vi "CRYAcq Get Channel Name.vi"(0 "I_channel Info Out":T2[](array[typedef]) {"Coupling" items=["Default"=-1, "RSE"=10083, "NRSE"=10078, "Differential"=10106, "Pseudodifferential"=12529]; "term config" items=["Default"=-1, "RSE"=10083, "NRSE"=10078, "Differential"=10106, "Pseudodifferential"=12529]; "Anti-aliasing Factor (%fs)" format="%.2f"}, 1 "O_channel Info Out":T2[](array[typedef]) {"Coupling" items=["Default"=-1, "RSE"=10083, "NRSE"=10078, "Differential"=10106, "Pseudodifferential"=12529]; "term config" items=["Default"=-1, "RSE"=10083, "NRSE"=10078, "Differential"=10106, "Pseudodifferential"=12529]; "Anti-aliasing Factor (%fs)" format="%.2f"}, 5 "Cluster":cluster{"RecDeviceID":u32, "Audio Driver":u32}, 9 "RecChannel":u16, 11 "Selected Play In":string[][](array[string]), 12 "Index for testinfor":i32, 13 "Acquisition Type":T1(ring)) -> (3 "Vmax In":dbl, 4 "ChannelName In":string caption="ChannelName", 6 "Test Info":string, 10 "Play Channel Name":string, 14 "In data Len":i32, 15 "Latency (samples) In":dbl)   [LabVIEW 2013]
uses:
  Typedef Control/CRYHardware Channel Info.ctl
panel:
  out "subarray":string[](array[string])
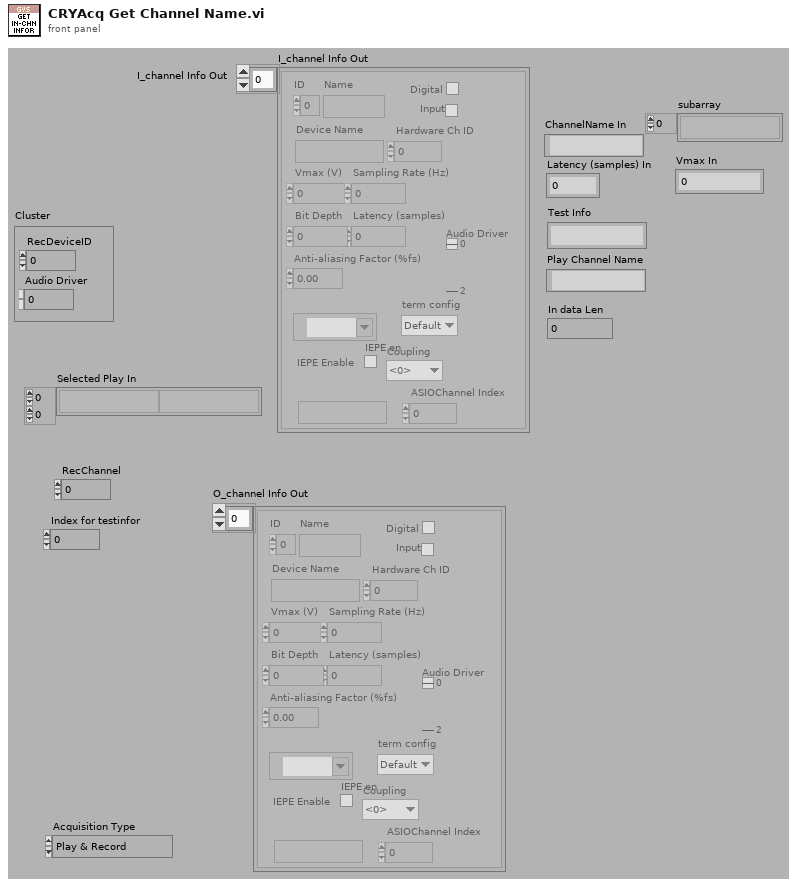
[diagram p1: front panel]
types:
  T1 = enum16{"Play & Record", "Record", "Sine Generator", "Voltmeter", "Oscilloscope", "Spectrum Analyzer", "RTA", "Generator & Voltmeter", "Generator & Oscilloscope", "Generator & Spectrum", "Generator & RTA"}
  T2 = typedef "CRYHardware Channel Info.ctl" = cluster{"ID":i32, "Name":string, "Digital":bool, "Input":bool, "Device Name":string, "Hardware Ch ID":u8, "Vmax (V)":dbl, "Latency (samples)":dbl, "Sampling Rate (Hz)":u32, "Bit Depth":u32, "Anti-aliasing Factor (%fs)":sgl, "DAQmx Channel":tag, "term config":i32, "Coupling":i32, "IEPE en":bool, "ASIOChannel Name":string, "Audio Driver":u16, "ASIOChannel Index":u8}
  T3 = typedef "CRYStimulus Test Infor Cluster.ctl" = cluster{"Stimulus Type":string, "Signal Type":string, "In/Out":bool, "FAPS":cluster{"freq":dbl, "ampl":dbl, "cycles":dbl, "samples":i32}[], "Sampling Rate":dbl, "Samples":i32, "Analysis Param":string, "Resolution":u16, "Steps":u32, "Analysis Value":dbl[], "Diff Freq":dbl, "FStart":dbl, "FStop":dbl, "Calibration Param":string, "Anti Alias":dbl, "Level Out1":dbl, "Level Out2":dbl, "EQ":bool}
  T4 = typedef "CRYWaveform Cluster.ctl" = cluster{"Waveform":cluster{"X0":dbl, "dX":dbl, "Y":sgl[]}, "X data":u16, "Y data":u16, "Y axis":u16, "X unit":string, "Y unit":string, "Y dB ref":dbl, "display Y":bool, "display X":bool, "Overload?":bool, "Test Info":string, "Step No.":i32, "Name":string, "protected":bool, "Sqc history":string[], "Signal Channel ID":i32, "Plot Settings":cluster{"Color":u32, "Interpolation":u8, "Point Style":u8, "Line Style":u8, "Point Color":u32, "Line Width":u8, "Bar Plot Style":u8, "Fill To":i16}, "AutoProtect":bool}
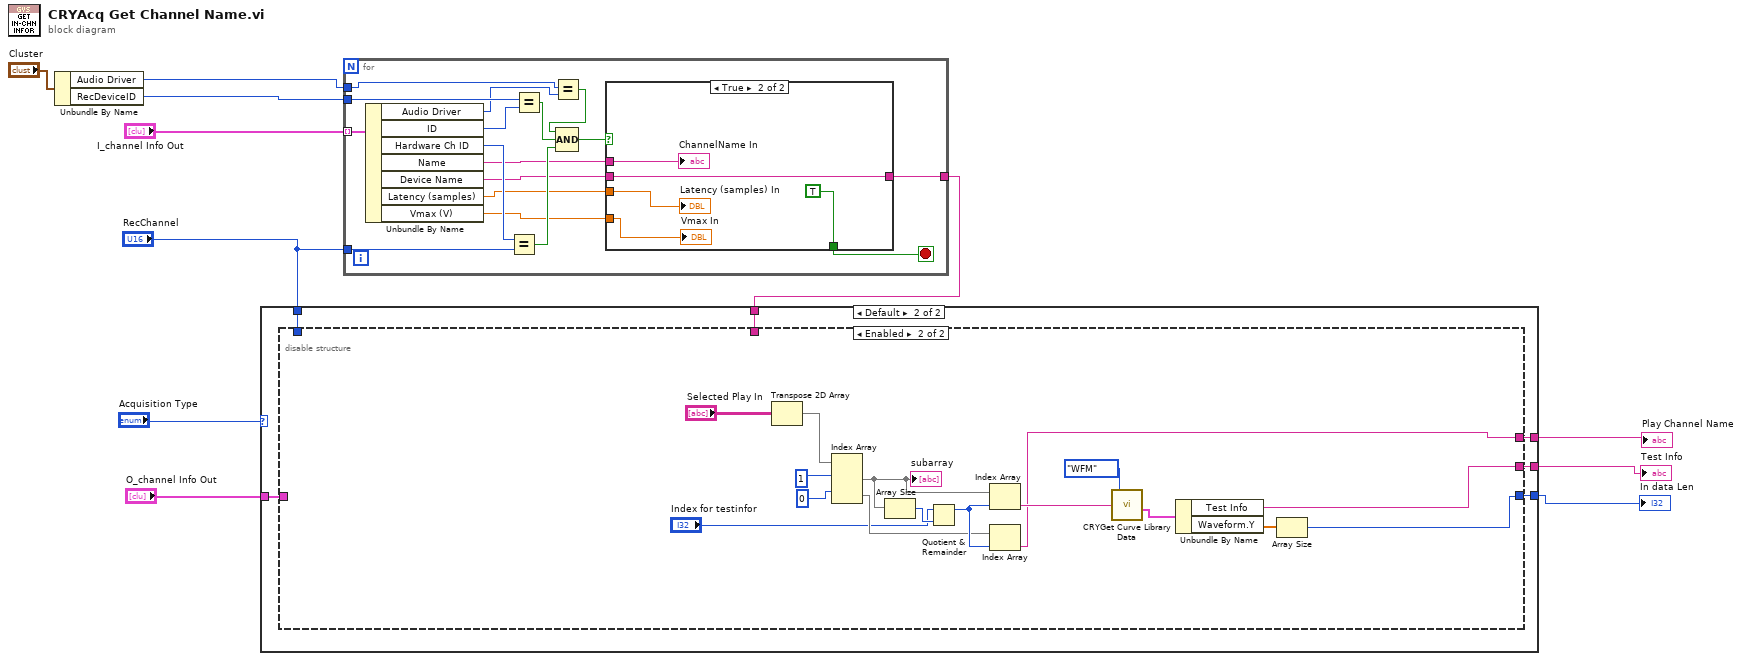
[diagram p0: block diagram]
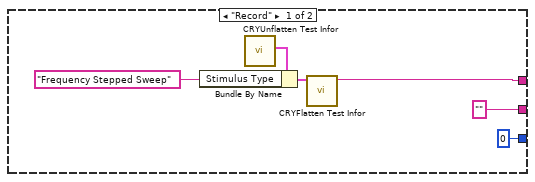
[diagram p2: hidden frame]
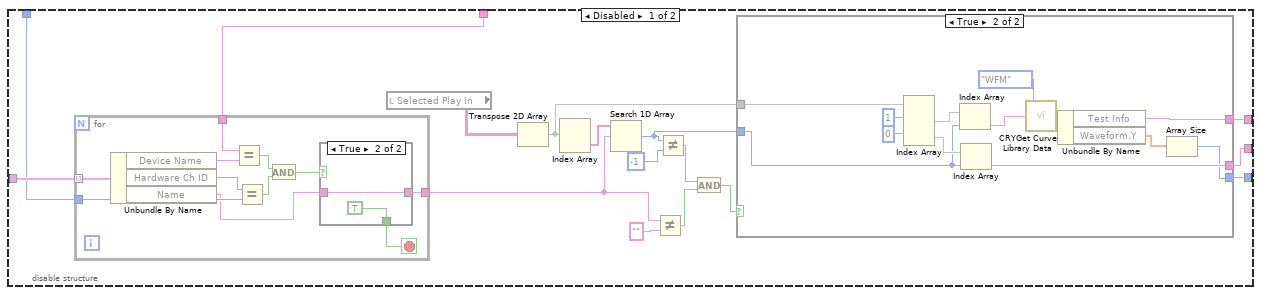
[diagram p3: hidden frame]
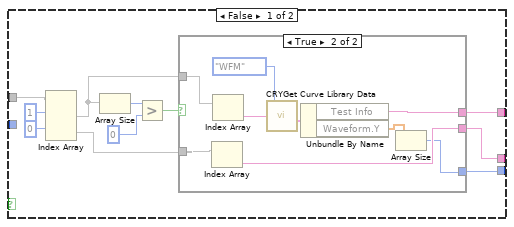
[diagram p4: hidden frame]
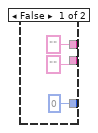
[diagram p5: hidden frame]
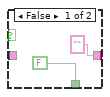
[diagram p6: hidden frame]
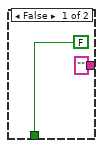
[diagram p7: hidden frame]
diagram:
  n1 = Unbundle By Name("Cluster") -> ("Audio Driver"=w6:u32, "RecDeviceID"=w7:u32)
  n2 = for {
    tunnel: "I_channel Info Out" -> [w28] mode=indexing
    tunnel: w7 -> [w27]
    tunnel: "RecChannel" -> [w24]
    tunnel: [w17] -> w4
    tunnel: w6 -> [w13]
    stop <- w19 stop-if-true
    n3 = Unbundle By Name(w28) -> ("Audio Driver"=w14:u16, "ID"=w26:i32, "Hardware Ch ID"=w25:u8, "Name"=w21:string, "Device Name"=w18:string, "Latency (samples)"=w16:dbl, "Vmax (V)"=w15:dbl)
    n4 = Equal?(x=w25, y=w24) -> (x = y?=w22:bool)
    n5 = Equal?(x=w27, y=w26) -> (x = y?=w23:bool)
    n6 = Equal?(x=w13, y=w14) -> (x = y?=w12:bool)
    n7 = Compound Arithmetic op=AND(w12, w23, w22) -> (w20:bool)
    n8 = case shown="True" w20 {
      tunnel: w21 -> [_ w35]
      tunnel: [FALSE TRUE] -> w19
      tunnel: w18 -> [_ w32]
      tunnel: ["" ("Device Name") w32] -> w17
      tunnel: w16 -> [_ w33]
      tunnel: w15 -> [_ w31]
      frame False {
      }
      frame True {
        "ChannelName In" <- w35
        "Latency (samples) In" <- w33
        "Vmax In" <- w31
      }
    }
  }
  n9 = case shown="Default" "Acquisition Type" {
    tunnel: "O_channel Info Out" -> [_ w47]
    tunnel: "RecChannel" -> [_ w46]
    tunnel: ["" ("Name") w45] -> w2
    tunnel: w4 -> [_ w44]
    tunnel: [w40 w43] -> w3
    tunnel: [0 w42] -> w1
    frame "Record" {
      n10 = call "CRYUnflatten Test Infor.vi"() -> ("unflattened test infor data"=w39:T3)  [unwired: 9 in, 1 out]
      n11 = Bundle By Name(cluster=w39, "Stimulus Type"="Frequency Stepped Sweep") -> (w37:T3)
      n12 = call "CRYFlatten Test Infor.vi"("Test Infor data"=w37) -> ("Fattened Data"=w40:string)  [unwired: 10 in]
    }
    frame Default {
      n13 = disable-structure shown="Enabled" {
        disable-tunnel: w47 -> [w63 _]
        disable-tunnel: w46 -> [w62 _]
        disable-tunnel: [w53 w117] -> w45
        disable-tunnel: w44 -> [w51 _]
        disable-tunnel: [w50 w116] -> w43
        disable-tunnel: [w49 w115] -> w42
        frame Disabled {
          n14 = for {
            tunnel: w63 -> [w110] mode=indexing
            tunnel: w62 -> [w108]
            tunnel: [w102] -> w52
            tunnel: w51 -> [w101]
            stop <- w103 stop-if-true
            n15 = Unbundle By Name(w110) -> ("Device Name"=w100:string, "Hardware Ch ID"=w109:u8, "Name"=w104:string)
            n16 = Equal?(x=w101, y=w100) -> (x = y?=w107:bool)
            n17 = Equal?(x=w109, y=w108) -> (x = y?=w106:bool)
            n18 = And(x=w107, y=w106) -> (x .and. y?=w105:bool)
            n19 = case shown="True" w105 {
              tunnel: w104 -> [_ w113]
              tunnel: [FALSE TRUE] -> w103
              tunnel: ["" ("Name") w113] -> w102
              frame False {
              }
              frame True {
              }
            }
          }
          n20 = local read "Selected Play In"() -> (w48:string[][])
          n21 = Transpose 2D Array(2D array=w48) -> (transposed array=w55:string[][])
          n22 = Index Array(array=w55) -> (element=w60:string[])  [unwired: 2 in]
          n23 = Search 1D Array(1D array=w60, element=w52) -> (index of element=w54:i32)  [unwired: 1 out]
          n24 = Not Equal?(x=w52, y="") -> (x != y?=w57:bool)
          n25 = Not Equal?(x=w54, y=-1) -> (x != y?=w58:bool)
          n26 = And(x=w58, y=w57) -> (x .and. y?=w56:bool)
          n27 = case shown="True" w56 {
            tunnel: w55 -> [w73 w99]
            tunnel: w54 -> [_ w90]
            tunnel: [w65 w94] -> w50
            tunnel: [w68 w89] -> w53
            tunnel: [w64 w87] -> w49
            frame False {
              n28 = Index Array(array=w73, index (row) #1=1 ("index (row)"), index (row) #2=0 ("index (row)")) -> (element #1=w69:string[], element #2=w66:string[])  [unwired: 2 in]
              n29 = Array Size(array=w69) -> (size(s)=w74:i32)
              n30 = Greater?(x=w74, y=0) -> (0:w70:bool)
              n31 = case shown="True" w70 {
                tunnel: w69 -> [_ w86]
                tunnel: ["" ("Test Info") w83] -> w65
                tunnel: ["" ("Test Info") w80] -> w68
                tunnel: w66 -> [_ w81]
                tunnel: [0 w78] -> w64
                frame False {
                }
                frame True {
                  n32 = Index Array(array=w81) -> (element=w80:string)  [unwired: 1 in]
                  n33 = Index Array(array=w86) -> (element=w82:string)  [unwired: 1 in]
                  n34 = call "CRYGet Curve Library Data.vi"("Type"=enum16{"Curves", "Values", "Results", "WFM"}."WFM", "Data Name"=w82) -> ("Wave"=w84:T4)  [unwired: 4 out]
                  n35 = Unbundle By Name(w84) -> ("Test Info"=w83:string, "Waveform.Y"=w79:sgl[])
                  n36 = Array Size(array=w79) -> (size(s)=w78:i32)
                }
              }
            }
            frame True {
              n37 = Index Array(array=w99, index (row) #1=1 ("index (row)"), index (row) #2=0 ("index (row)")) -> (element #1=w97:string[], element #2=w91:string[])  [unwired: 2 in]
              n38 = Index Array(array=w97, index=w90) -> (element=w93:string)
              n39 = Index Array(array=w91, index=w90) -> (element=w89:string)
              n40 = call "CRYGet Curve Library Data.vi"("Type"=enum16{"Curves", "Values", "Results", "WFM"}."WFM", "Data Name"=w93) -> ("Wave"=w95:T4)  [unwired: 4 out]
              n41 = Unbundle By Name(w95) -> ("Test Info"=w94:string, "Waveform.Y"=w88:sgl[])
              n42 = Array Size(array=w88) -> (size(s)=w87:i32)
            }
          }
        }
        frame Enabled {
          n43 = Transpose 2D Array(2D array="Selected Play In") -> (transposed array=w124:string[][])
          n44 = Index Array(array=w124, index (row) #1=1 ("index (row)"), index (row) #2=0 ("index (row)")) -> (element #1=w127:string[], element #2=w128:string[])  [unwired: 2 in]
          "subarray" <- w127
          n45 = Array Size(array=w127) -> (size(s)=w119:i32)
          n46 = Quotient & Remainder(x="Index for testinfor", y=w119) -> (x-y*floor(x/y)=w129:i32)  [unwired: 1 out]
          n47 = Index Array(array=w127, index=w129) -> (element=w123:string)
          n48 = Index Array(array=w128, index=w129) -> (element=w116:string)
          n49 = call "CRYGet Curve Library Data.vi"("Type"=enum16{"Curves", "Values", "Results", "WFM"}."WFM", "Data Name"=w123) -> ("Wave"=w121:T4)  [unwired: 4 out]
          n50 = Unbundle By Name(w121) -> ("Test Info"=w117:string, "Waveform.Y"=w120:sgl[])
          n51 = Array Size(array=w120) -> (size(s)=w115:i32)
        }
      }
    }
  }
  "Play Channel Name" <- w3
  "Test Info" <- w2
  "In data Len" <- w1
